vi "Process Mouse Move.vi"(10 "Coords":T4, 11 "Core Data in":T1) -> (3 "Core Data out":T1)   [LabVIEW 2020, in "Amnesia.lvlib"]
uses:
  Amnesia.lvlib
  Rotating Objects/Rotating Objects.lvclass
  C:/dev/LabGame/Source/Scene/Scene.lvclass
  Scene/Scene.lvclass/Scene.ctl
  Scene/Scene.lvclass
  <vilib>/Utility/miscctls.llb/LVPoint32TypeDef.ctl
  Core Data.ctl
  Scene/Mouse Button Held.ctl
  <vilib>/Dataflow_G/G-Audio/Controls/Audio Device Refnum.ctl
  <vilib>/Dataflow_G/G-Audio/G-Audio.lvlib
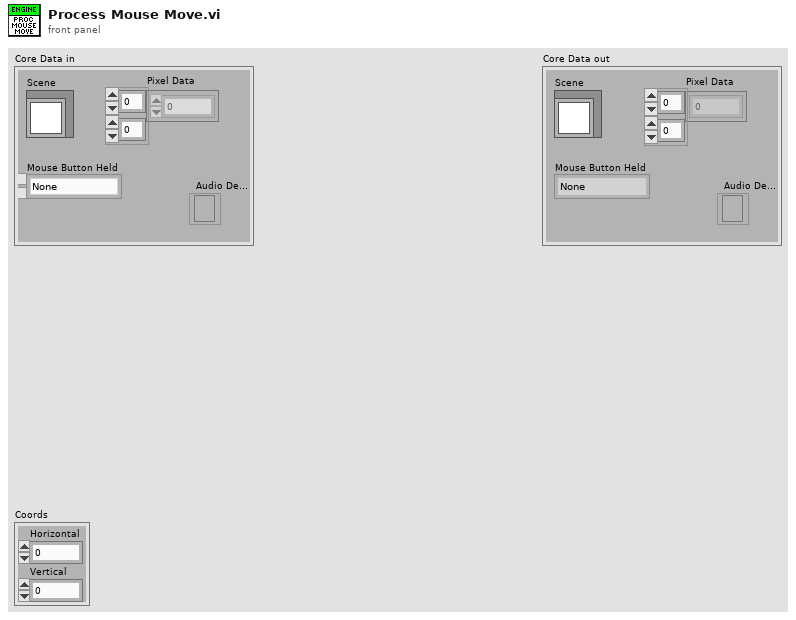
[diagram p1: front panel]
types:
  T1 = typedef "Amnesia.lvlib/Core Data.ctl" = cluster{"Pixel Data":u32[][], "Scene":refnum<class "Rotating Objects.lvclass">, "Mouse Button Held":T2, "Audio Device":T3}
  T2 = typedef "Scene.lvclass/Mouse Button Held.ctl" = enum16{"None", "Left", "Middle", "Right"}
  T3 = typedef "G-Audio.lvlib/Audio Device Refnum.ctl" = refnum<file>
  T4 = typedef "LVPoint32TypeDef.ctl" = cluster{"Horizontal":i32, "Vertical":i32}
  T5 = typedef "3D.lvlib/Transform.ctl" = cluster{"Position":T6, "Rotation":T6, "Scale":T6}
  T6 = typedef "3D.lvlib/Vector 3D.ctl" = cluster{"x":sgl, "y":sgl, "z":sgl}
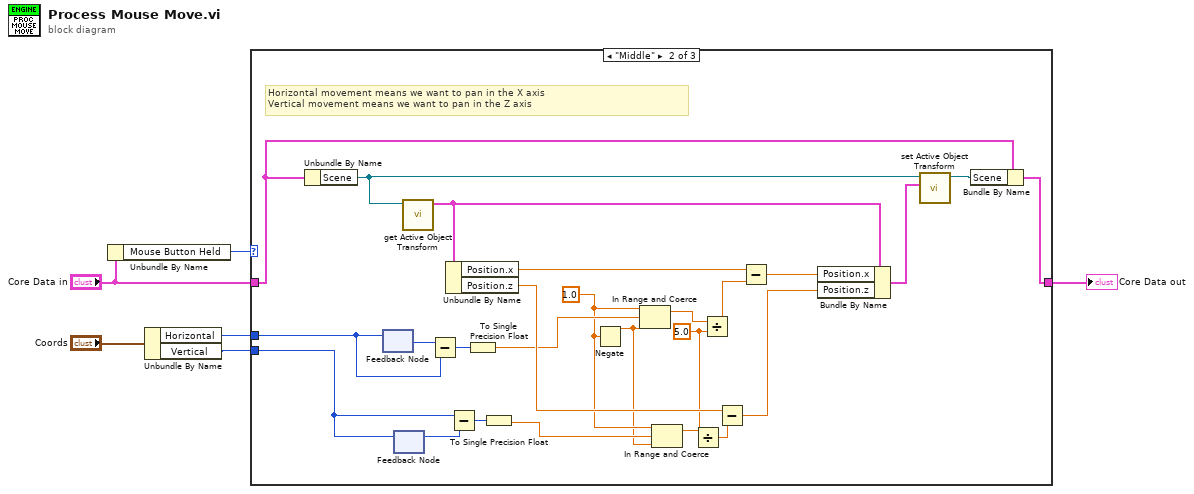
[diagram p0: block diagram]
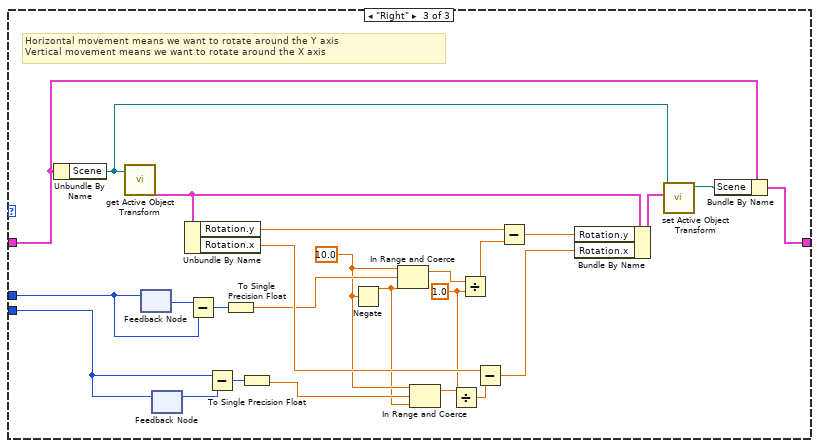
[diagram p3: hidden frame]
diagram:
  n1 = Unbundle By Name("Core Data in") -> ("Mouse Button Held"=w3:T2)
  n2 = Unbundle By Name("Coords") -> ("Horizontal"=w2:i32, "Vertical"=w1:i32)
  n3 = case shown="\"Middle\"" w3 {
    tunnel: [w7 w10 w33] -> w5
    tunnel: w2 -> [_ w30 w55]
    tunnel: "Core Data in" -> [w7 w11 w34]
    tunnel: w1 -> [_ w23 w48]
    frame "None", Default {
    }
    frame "Middle" {
      w14 = sgl 5.0 ("y")
      w20 = sgl 1.0 ("upper limit")
      # "Horizontal movement means we want to pan in the X axis\nVertical movement means we want to pan in the Z axis"
      n4 = Unbundle By Name(w11) -> ("Scene"=w12:refnum<class "Rotating Objects.lvclass">)
      n5 = feedback #1() -> (w29:i32)  [unwired: 1 in]
      n6 = feedback-in #1(w30) -> ()
      n7 = feedback #2() -> (w28:i32)  [unwired: 1 in]
      n8 = feedback-in #2(w23) -> ()
      n9 = call "get Active Object Transform.vi"("Scene in"=w12) -> ("Transform"=w13:T5)  [unwired: 10 in]
      n10 = Subtract(x=w29, y=w30) -> (x-y=w25:i32)
      n11 = Unbundle By Name(w13) -> ("Position.x"=w32:sgl, "Position.z"=w27:sgl)
      n12 = Subtract(x=w23, y=w28) -> (x-y=w24:i32)
      n13 = To Single Precision Float(number=w25) -> (single precision float=w22:sgl)
      n14 = To Single Precision Float(number=w24) -> (single precision float=w21:sgl)
      n15 = Negate(x=w20) -> (-x=w19:sgl)
      n16 = In Range and Coerce(upper limit=w20, x=w22, lower limit=w19) -> (coerced(x)=w18:sgl)  [unwired: 1 out]
      n17 = In Range and Coerce(upper limit=w20, x=w21, lower limit=w19) -> (coerced(x)=w16:sgl)  [unwired: 1 out]
      n18 = Divide(x=w16, y=w14) -> (x/y=w15:sgl)
      n19 = Divide(x=w18, y=w14) -> (x/y=w17:sgl)
      n20 = Subtract(x=w27, y=w15) -> (x-y=w26:sgl)
      n21 = Subtract(x=w32, y=w17) -> (x-y=w31:sgl)
      n22 = Bundle By Name(cluster=w13, "Position.x"=w31, "Position.z"=w26) -> (w8:T5)
      n23 = call "set Active Object Transform.vi"("Transform"=w8, "Scene in"=w12) -> ("Scene out"=w9:refnum<class "Rotating Objects.lvclass">)  [unwired: 9 in]
      n24 = Bundle By Name(cluster=w11, "Scene"=w9) -> (w10:T1)
    }
    frame "Right" {
      w39 = sgl 1.0 ("y")
      w45 = sgl 10.0 ("upper limit")
      # "Horizontal movement means we want to rotate around the Y axis\nVertical movement means we want to rotate around the X axis"
      n25 = Unbundle By Name(w34) -> ("Scene"=w37:refnum<class "Rotating Objects.lvclass">)
      n26 = call "get Active Object Transform.vi"("Scene in"=w37) -> ("Transform"=w36:T5)  [unwired: 10 in]
      n27 = feedback #3() -> (w54:i32)  [unwired: 1 in]
      n28 = feedback-in #3(w55) -> ()
      n29 = feedback #4() -> (w53:i32)  [unwired: 1 in]
      n30 = feedback-in #4(w48) -> ()
      n31 = Unbundle By Name(w36) -> ("Rotation.y"=w57:sgl, "Rotation.x"=w52:sgl)
      n32 = Subtract(x=w54, y=w55) -> (x-y=w50:i32)
      n33 = Subtract(x=w48, y=w53) -> (x-y=w49:i32)
      n34 = To Single Precision Float(number=w50) -> (single precision float=w47:sgl)
      n35 = To Single Precision Float(number=w49) -> (single precision float=w46:sgl)
      n36 = Negate(x=w45) -> (-x=w44:sgl)
      n37 = In Range and Coerce(upper limit=w45, x=w47, lower limit=w44) -> (coerced(x)=w43:sgl)  [unwired: 1 out]
      n38 = In Range and Coerce(upper limit=w45, x=w46, lower limit=w44) -> (coerced(x)=w41:sgl)  [unwired: 1 out]
      n39 = Divide(x=w41, y=w39) -> (x/y=w40:sgl)
      n40 = Divide(x=w43, y=w39) -> (x/y=w42:sgl)
      n41 = Subtract(x=w52, y=w40) -> (x-y=w51:sgl)
      n42 = Subtract(x=w57, y=w42) -> (x-y=w56:sgl)
      n43 = Bundle By Name(cluster=w36, "Rotation.y"=w56, "Rotation.x"=w51) -> (w35:T5)
      n44 = call "set Active Object Transform.vi"("Transform"=w35, "Scene in"=w37) -> ("Scene out"=w38:refnum<class "Rotating Objects.lvclass">)  [unwired: 9 in]
      n45 = Bundle By Name(cluster=w34, "Scene"=w38) -> (w33:T1)
    }
  }
  "Core Data out" <- w5
